vi "Pre-Process and HU Validation.vi"(8 "error in":errorcluster, 11 "Input Parameters":T2) -> (0 "error out":errorcluster, 3 "Output Parameetrs":T1)   [LabVIEW 2023]
doc: "With this VI it is check if device can be tested on station. All fields are required. Example :\nOperator = 0043, SerialNo = 3144369-AA01S251219OK02, MaterialCode = 604-003-00-00.\nPossible Errors : Serial Number and material code missmatch, Previous process failure, Previous process skipped and Already packed in HU [400000355]"
uses:
  <userlib>/WebService/_CheckPqmNtrsAndProductSerialDateService/CheckPqmNtrsAndProductSerialDateService.lvlib
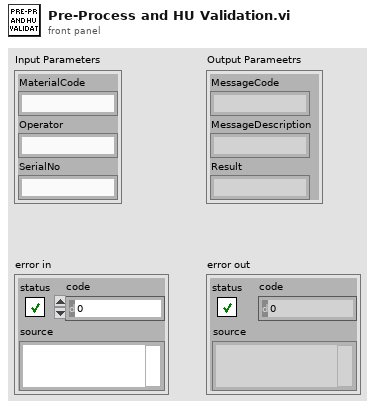
[diagram p1: front panel]
types:
  T1 = cluster{"MessageCode":string, "MessageDescription":string, "Result":string}
  T2 = cluster{"MaterialCode":string, "Operator":string, "SerialNo":string}
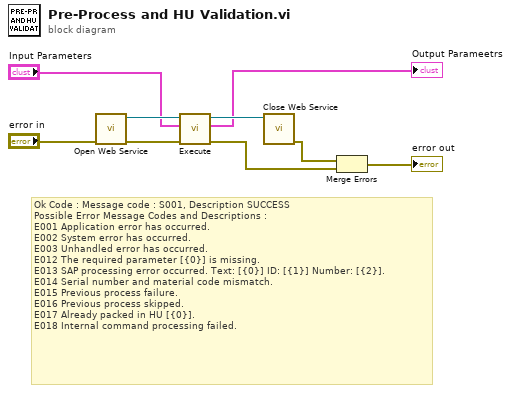
[diagram p0: block diagram]
diagram:
  # "Ok Code : Message code : S001, Description SUCCESS \nPossible Error Message Codes and Descriptions :\nE001 Application error has occurred.\nE002 System error has occurred.\nE003 Unhandled error has occurred.\nE012 The required parameter [{0}] is missing. \nE013 SAP processing error occurred. Text: [{0}] ID: [{1}] Number: [{2}].\nE014 Serial number and material code mismatch.\nE015 Previous process failure.\nE016 Previous process skipped.\nE017 Already packed in HU [{0}].\nE018 Internal command processing failed."
  n1 = call <userlib>:"Open Web Service.vi"("error in (no error)"="error in") -> ("error out"=w8:errorcluster, "CheckPqmNtrsAndProductSerialDateService refnum"=w4:refnum<k24>)  [unwired: 9 in]
  n2 = call <userlib>:"Execute.vi"("error in (no error)"=w8, ".NET:CheckPqmNtrsAndProductSerialDateService.PqmNtrsAndProductSerialRequest"="Input Parameters", "CheckPqmNtrsAndProductSerialDateService refnum"=w4) -> ("error out"=w7:errorcluster, ".NET:CheckPqmNtrsAndProductSerialDateService.CommonResponse"=→"Output Parameetrs":T1, "CheckPqmNtrsAndProductSerialDateService refnum out"=w3:refnum<k24>)  [unwired: 6 in]
  n3 = call <userlib>:"Close Web Service.vi"("CheckPqmNtrsAndProductSerialDateService refnum"=w3) -> ("error out"=w6:errorcluster)  [unwired: 10 in]
  n4 = Merge Errors(w6, w7) -> (→"error out":errorcluster)
